vi "_Wait for axes to stop.vi"(0 "System no.":i32=1, 2 "Axes to wait for":string[](array[string]), 3 "With status bit polling?":bool, 5 "error in":errorcluster, 7 "Polling cycle time, ms":u32=400, 12 "Stop refnum":refnum<vi>) -> (14 "Stopped":bool, 19 "error out":errorcluster)   [LabVIEW 2014]
doc: "This VI waits for the specified axes to stop using #5 polling. It also stops if a communication error occured, Stop refnum or Local stop is TRUE. Requires \"STA?.vi\" to be present. Required by \"General wait for movement to stop.vi\". When using as a sub-VI, use Stop refnum to stop VI from caller.\n\nValid for C-702, C-843, C-843.PM, C-844, C-848, C-865, C-867, C-880, E-517, E-712, E-725, E-753, E-755, E-861, Mercury™ (but must be present in Support.llb for all other systems also)\n\nC-880: With status bit polling? = TRUE\n\nAll other systems: With status bit polling? = FALSE"
panel:
  in  "Local stop":bool
  # "This vi waits for the specified axes to stop using #5 polling. \nIt also stops if a communications error occured, Stop refnum\nor Local stop is TRUE."
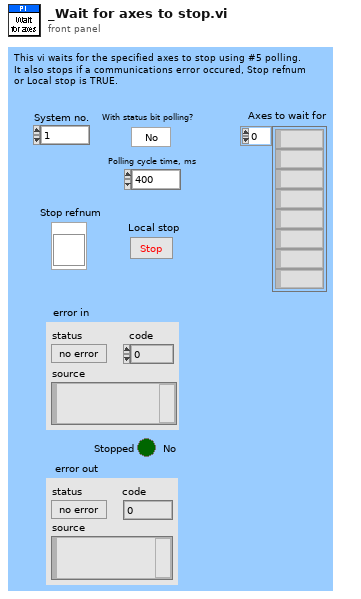
[diagram p1: front panel]
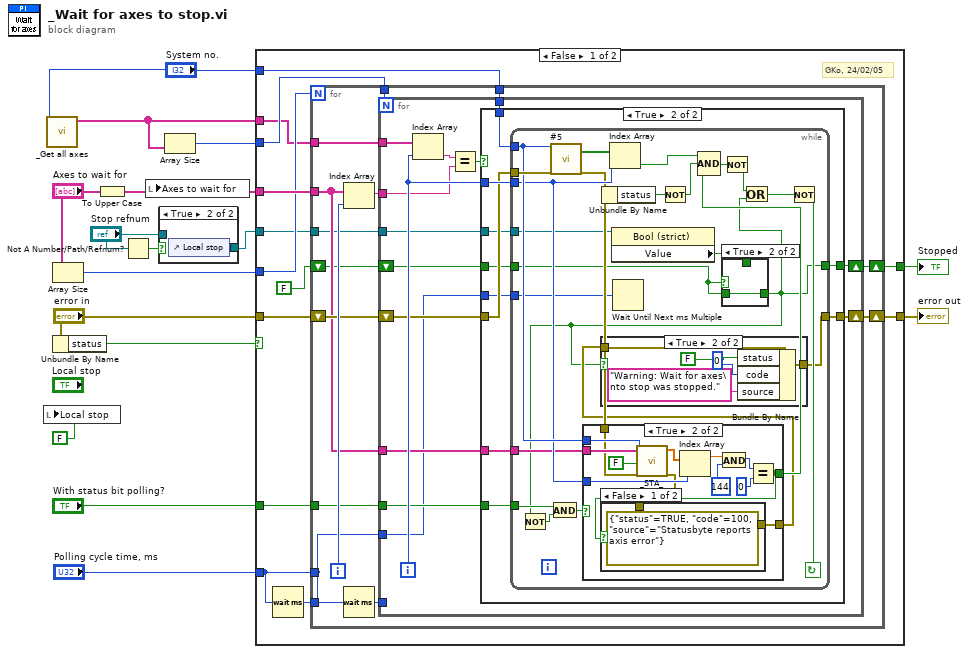
[diagram p0: block diagram]
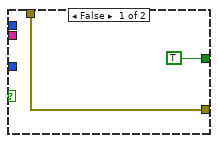
[diagram p6: hidden frame]
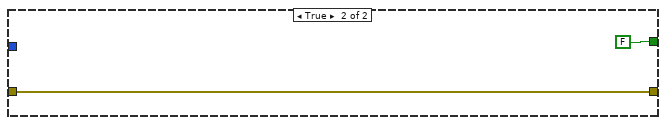
[diagram p8: hidden frame]
diagram:
  n1 = local write "Local stop"(FALSE ("Local stop")) -> ()
  n2 = call "_Get all axes.vi"("System no."="System no.") -> ("Conn. Axes"=w2:string[])  [unwired: 18 in]
  n3 = Array Size(array="Axes to wait for") -> (size(s)=w12:i32)
  n4 = Unbundle By Name("error in") -> ("status"=w14:bool)
  n5 = To Upper Case(1:"Axes to wait for") -> (0:w10:string[])
  n6 = Not A Number/Path/Refnum?(number/path/refnum="Stop refnum") -> (NaN/Path/Refnum?=w5:bool)
  n7 = local write "Axes to wait for"(w10) -> ()
  n8 = case shown="True" w5 {
    tunnel: [w17 w18] -> w4
    tunnel: "Stop refnum" -> [w17 _]
    frame False {
    }
    frame True {
      n9 = control-ref of="Local stop"() -> (w18:refnum<vi>)
    }
  }
  n10 = Array Size(array=w2) -> (size(s)=w13:i32)
  n11 = case shown="False" w14 {
    tunnel: "System no." -> [w31 _]
    tunnel: w2 -> [w26 _]
    tunnel: w13 -> [w30 _]
    tunnel: w10 -> [w29 _]
    tunnel: w12 -> [w28 _]
    tunnel: "error in" -> [w27 w122]
    tunnel: [w25 w122] -> w11
    tunnel: "With status bit polling?" -> [w24 _]
    tunnel: "Polling cycle time, ms" -> [w23 _]
    tunnel: w4 -> [w21 _]
    tunnel: [w19 FALSE ("Value")] -> w3
    frame False {
      # "GKo, 24/02/05"
      n12 = Wait (ms)(milliseconds to wait=w23) -> (millisecond timer value=w22:u32)
      n13 = for {
        N: w28 -> [_]
        tunnel: w29 -> [w36]
        tunnel: w30 -> [w44]
        tunnel: w31 -> [w42]
        shift-right: [w40] -> w25
        shift-left: w27 -> [w41]
        tunnel: w26 -> [w39]
        tunnel: w24 -> [w38]
        tunnel: w23 -> [w35]
        tunnel: w22 -> [_]
        tunnel: w21 -> [w34]
        shift-right: [w32] -> w19
        shift-left: FALSE -> [w33]
        i -> [w45]
        n14 = Index Array(array=w36, index=w45) -> (element=w43:string)
        n15 = Wait (ms)(milliseconds to wait=w35) -> (millisecond timer value=w37:u32)
        n16 = for {
          N: w44 -> [_]
          tunnel: w43 -> [w52]
          tunnel: w42 -> [w57]
          shift-right: [w54] -> w40
          shift-left: w41 -> [w55]
          tunnel: w39 -> [w51]
          tunnel: w38 -> [w53]
          tunnel: w37 -> [_]
          tunnel: w36 -> [w50]
          tunnel: w35 -> [w49]
          tunnel: w34 -> [w48]
          shift-right: [w46] -> w32
          shift-left: w33 -> [w47]
          i -> [w56]
          n17 = Index Array(array=w51, index=w56) -> (element=w59:string)
          n18 = Equal?(x=w59, y=w52) -> (x = y?=w58:bool)
          n19 = case shown="True" w58 {
            tunnel: w57 -> [_ w71]
            tunnel: w56 -> [_ w70]
            tunnel: w55 -> [w61 w69]
            tunnel: [w61 w67] -> w54
            tunnel: w53 -> [_ w68]
            tunnel: w50 -> [_ w66]
            tunnel: w49 -> [_ w65]
            tunnel: w48 -> [_ w64]
            tunnel: [w60 w63] -> w46
            tunnel: w47 -> [w60 w62]
            frame False {
            }
            frame True {
              n20 = while {
                tunnel: w62 -> [w74]
                tunnel: [w72] -> w63
                tunnel: w64 -> [w75]
                tunnel: w65 -> [w85]
                tunnel: w66 -> [w87]
                tunnel: [w80] -> w67
                tunnel: w68 -> [w78]
                tunnel: w69 -> [w91]
                tunnel: w70 -> [w89]
                tunnel: w71 -> [w90]
                stop <- w81 continue-if-true
                n21 = call "#5.vi"("System no."=w90, "error in"=w91) -> ("Axis moving?"=w95:bool[], "error out"=w88:errorcluster)  [unwired: 16 in]
                n22 = Unbundle By Name(w88) -> ("status"=w94:bool)
                n23 = Index Array(array=w95, index=w89) -> (element=w92:bool)
                n24 = property class="Bool (strict)"(reference=w75) -> ("Value"=w73:bool)  [unwired: 1 in, 2 out]
                n25 = Wait Until Next ms Multiple(millisecond multiple=w85) -> ()  [unwired: 1 out]
                n26 = Not(x=w94) -> (.not. x?=w93:bool)
                n27 = case shown="True" w74 {
                  tunnel: [w96 w97] -> w72
                  tunnel: w74 -> [_ w97]
                  tunnel: w73 -> [w96 _]
                  frame False {
                  }
                  frame True {
                  }
                }
                n28 = Not(x=w72) -> (.not. x?=w76:bool)
                n29 = And(x=w78, y=w76) -> (x .and. y?=w77:bool)
                n30 = case shown="True" w77 {
                  tunnel: w90 -> [_ w118]
                  tunnel: w89 -> [_ w116]
                  tunnel: w88 -> [w105 w114]
                  tunnel: [w105 w108] -> w79
                  tunnel: w87 -> [_ w115]
                  tunnel: [TRUE w107] -> w86
                  frame False {
                  }
                  frame True {
                    n31 = call "_STA_.vi"("System no."=w118, "Axes to query"=w115, "All axes?"=FALSE, "error in"=w114) -> ("Axis status"=w117:dbl[], "error out"=w106:errorcluster)  [unwired: 14 in]
                    n32 = Index Array(array=w117, index=w116) -> (element=w112:dbl)
                    n33 = And(x=w112, y=u32 144) -> (x .and. y?=w110:i32)
                    n34 = Equal?(x=w110, y=0) -> (x = y?=w107:bool)
                    n35 = case shown="False" w107 {
                      tunnel: [errorcluster {"status"=TRUE, "code"=100, "source"="Statusbyte reports axis error"} ("error out") w120] -> w108
                      tunnel: w106 -> [_ w120]
                      frame False {
                      }
                      frame True {
                      }
                    }
                  }
                }
                n36 = case shown="True" w72 {
                  tunnel: [w98 w102] -> w80
                  tunnel: w79 -> [w98 w103]
                  frame False {
                  }
                  frame True {
                    n37 = Bundle By Name(cluster=w103, "status"=FALSE, "code"=0, "source"="Warning: Wait for axes\nto stop was stopped.") -> (w102:errorcluster)
                  }
                }
                n38 = Compound Arithmetic op=AND(w92, w93, w86) -> (w84:bool)
                n39 = Not(x=w84) -> (.not. x?=w83:bool)
                n40 = Or(x=w83, y=w72) -> (x .or. y?=w82:bool)
                n41 = Not(x=w82) -> (.not. x?=w81:bool)
              }
            }
          }
        }
      }
    }
    frame True {
    }
  }
  "error out" <- w11
  "Stopped" <- w3
